vi "Send Tree Edit Cell.vi"(4 "Col":i32, 5 "EventFilter Reference":T1, 6 "Tag":string, 8 "String":string, 9 "Time":u32, 10 "CtlRef":refnum<vi>, 11 "Message Enqueuer in":refnum<class "Message Enqueuer.lvclass">) -> (0 "error out":errorcluster, 3 "Filtered EventDataMessage":refnum<class "TreeEditCellMsg.lvclass">)   [LabVIEW 2015, in "ActorEvents.lvlib" / "TreeEditCellMsg.lvclass"]
doc: "<License>\nCopyright © 2017 Composed Systems, LLC | All rights reserved\nwww.composed.io\n\nAuthor: Ethan Stern <ethan.stern@composed.io>\n\nThis software is provided \"AS IS\" WITHOUT WARRANTIES, either express or implied, AND IS FOR EDUCATIONAL PURPOSES ONLY.\n</License>"
uses:
  TreeEditCellMsg.lvclass
  <vilib>/ActorFramework/Message Enqueuer/Message Enqueuer.lvclass
  IEventFilter/EventFilter Reference.ctl
  IEventFilter/IEventFilter.lvclass
  TreeEditCellMsg.lvclass/TreeEditCellMsg.ctl
  EventDataMessage/EventDataMessage.lvclass/EventDataMessage.ctl
  <vilib>/ActorFramework/Message Enqueuer/Message Enqueuer.lvclass/Message Enqueuer.ctl
  <vilib>/ActorFramework/Message Enqueuer/Enqueue.vi
  <vilib>/Utility/error.llb/Clear Errors.vi
  <vilib>/ActorFramework/Message Priority Queue/Priority Enqueue.vi
  EventDataMessage/EventDataMessage.lvclass
panel:
  in  "error in (no error)":errorcluster
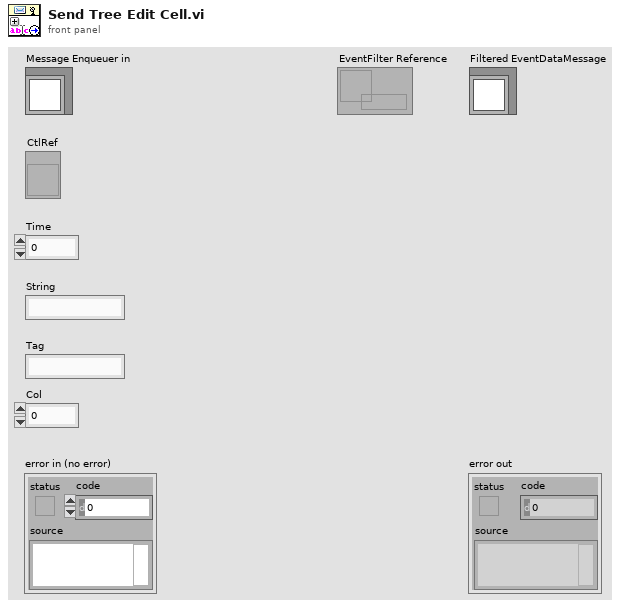
[diagram p1: front panel]
types:
  T1 = typedef "ActorEvents.lvlib/IEventFilter.lvclass/EventFilter Reference.ctl" = refnum<data-value>
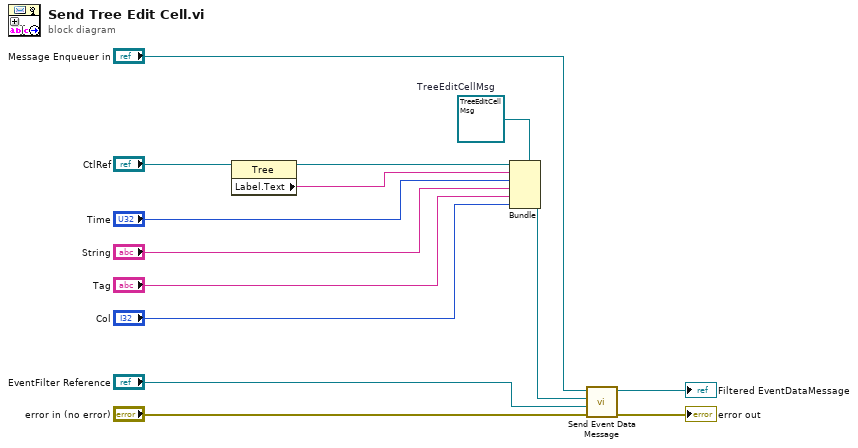
[diagram p0: block diagram]
diagram:
  w14 = refnum<class "TreeEditCellMsg.lvclass"> refnum  # TreeEditCellMsg
  n1 = property class="Tree"(reference="CtlRef") -> (reference out=w8:refnum<vi>, "Label.Text"=w3:string)  [unwired: 1 in, 1 out]
  n2 = Bundle(cluster=w14, w8, w3, "Time", "String", "Tag", "Col") -> (w11:refnum<class "TreeEditCellMsg.lvclass">)
  n3 = call "Send Event Data Message.vi"("error in (no error)"="error in (no error)", "EventFilter Reference"="EventFilter Reference", "EventDataMessage"=w11, "Message Enqueuer in"="Message Enqueuer in") -> ("error out"=→"error out":errorcluster, "Filtered EventDataMessage"=→"Filtered EventDataMessage":refnum<class "TreeEditCellMsg.lvclass">)  [unwired: 6 in]
